vi "Low level.vi"() -> ()   [LabVIEW 2011, in "Diamond Universal Driver.lvlib"]
uses:
  Diamond Universal Driver.lvlib
panel:
  out "x+y":i32 format="%x"
  in  "Boolean array 2":bool[](array[boolean])
  out "error out":errorcluster
  out "Boolean array":bool[](array[boolean])
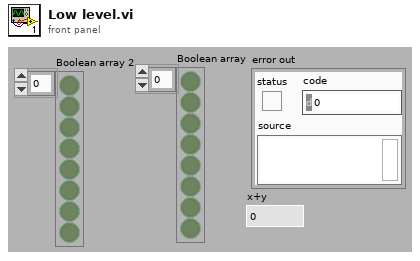
[diagram p1: front panel]
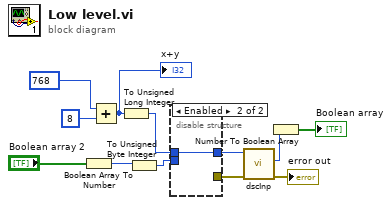
[diagram p0: block diagram]
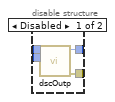
[diagram p2: hidden frame]
diagram:
  n1 = Boolean Array To Number(Boolean array="Boolean array 2") -> (number=w6:u32)
  n2 = Add(x=768, y=8) -> (x+y=w10:i32)
  "x+y" <- w10
  n3 = To Unsigned Long Integer(number=w10) -> (unsigned 32bit integer=w8:u32)
  n4 = To Unsigned Byte Integer(number=w6) -> (unsigned 8bit integer=w1:u8)
  n5 = disable-structure shown="Enabled" {
    disable-tunnel: w8 -> [w16 w17]
    disable-tunnel: [w15 w17] -> w5
    disable-tunnel: [w14 _] -> w4
    disable-tunnel: w1 -> [w13 _]
    frame Disabled {
      n6 = call "dscOutp.vi"("valueIn"=w13, "addressIn"=w16) -> ("error out"=w14:errorcluster, "addressOut"=w15:u32)  [unwired: 7 in, 1 out]
    }
    frame Enabled {
    }
  }
  n7 = call "dscInp.vi"("error in"=w4, "addressIn"=w5) -> ("error out"=→"error out":errorcluster, "value"=w3:u8)  [unwired: 7 in, 1 out]
  n8 = Number To Boolean Array(number=w3) -> (Boolean array=→"Boolean array":bool[])
